vi "Sr830 Write Param.vi"(6 "Time Constant":u16(ring)=1 items=["10 us", "30 us", "100 us", "300 us", "1 ms", "3 ms", "10 ms", "30 ms", "100 ms", "300 ms", "1 s", "3 s", "10 s", "30 s", "100 s", "300 s", "1 ks", "3 ks", "10 ks", "30 ks"], 7 "Dynamic Reserve":u16(ring) items=["High", "Normal", "Low"], 8 "error in":errorcluster, 9 "Sensitivity":u16(ring)=1 items=["2 nV/fA", "5 nV/fA", "10 nV/fA", "20 nV/fA", "50 nV/fA", "100 nV/fA", "200 nV/fA", "500 nV/fA", "1 µV/pA", "2 µV/pA", "5 µV/pA", "10 µV/pA", "20 µV/pA", "50 µV/pA", "100µV/pA", "200 µV/pA", "500µV/pA", "1 mV/nA", "2 mV/nA", "5 mV/nA", "10 mV/nA", "20 mV/nA", "50 mV/nA", "100 mV/nA", "200 mV/nA", "500 mV/nA", "1 V/uA"], 10 "Param":T1(ring), 11 "Ressource VISA":refnum<visa-resource-name>="GPIB0::8::INSTR") -> (0 "error out":errorcluster, 3 "Ressource VISA Out":refnum<visa-resource-name>="GPIB0::8::INSTR")   [LabVIEW 2019]
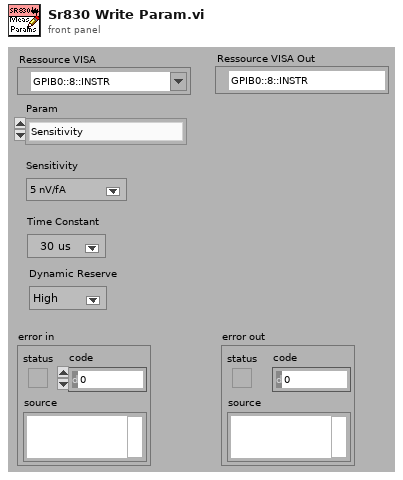
[diagram p1: front panel]
types:
  T1 = enum16{"Sensitivity", "Dynamic Reserve", "Time Constant"}
  T2 = enum16{"Phase Shift", "Reference Source", "Reference Frequency", "Reference Trigger", "Detection Harmonic", "Sine Amplitude", "Input Configuration", "Input Shield", "Input Coupling", "Input Line Notch Filter", "Sensitivity", "Dynamic Reserve", "Time Constant", "Low Pass Filter", "Sync Filter", "Expand X", "Expand Y", "Expand R", "All"}
  T3 = cluster{"Phase Shift (°)":dbl, "Reference Source":u16, "Frequency (Hz)":dbl, "Reference Trigger":u16, "Harmonic":i32, "Sine Amplitude (V)":dbl, "Input Configuration":u16, "Input Shield":u16, "Input Coupling":u16, "Input Notch Filters":cluster{"1xLineFilter":bool, "2xLineFilter":bool}, "Sensitivity":u16, "Dynamic Reserve":u16, "Time Constant":u16, "Low Pass Filter":u16, "Sync Filter":bool, "Expand X":cluster{"Offset (%)":dbl, "Expand":u16}, "Expand Y":cluster{"Offset (%)":dbl, "Expand":u16}, "Expand R":cluster{"Offset (%)":dbl, "Expand":u16}}
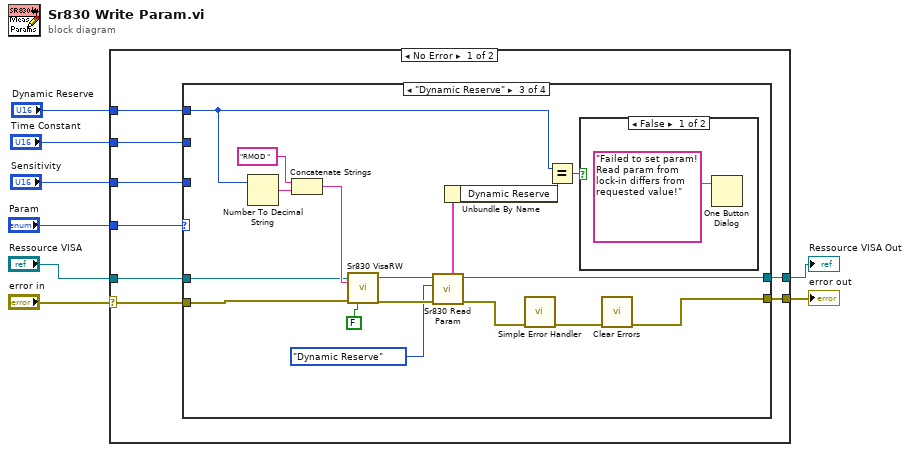
[diagram p0: block diagram]
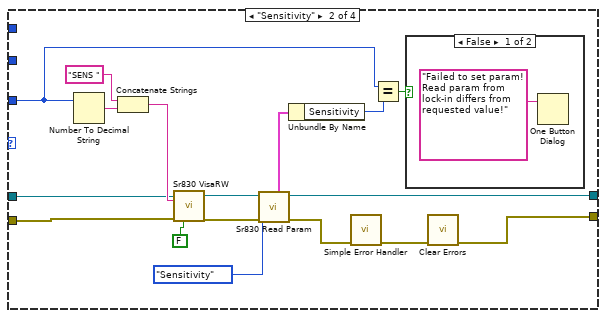
[diagram p3: hidden frame]
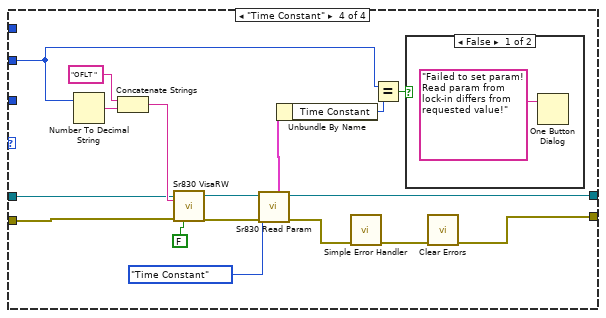
[diagram p6: hidden frame]
diagram:
  n1 = case shown="No Error" "error in" {
    selector: "error in" -> [w14 w74]
    tunnel: [w15 w74] -> w8
    tunnel: "Ressource VISA" -> [w13 w73]
    tunnel: [w16 w73] -> w5
    tunnel: "Sensitivity" -> [w12 _]
    tunnel: "Param" -> [w11 _]
    tunnel: "Dynamic Reserve" -> [w10 _]
    tunnel: "Time Constant" -> [w9 _]
    frame No Error {
      n2 = case shown="\"Dynamic Reserve\"" w11 {
        tunnel: [w17 w21 w40 w58] -> w16
        tunnel: [w18 w19 w38 w56] -> w15
        tunnel: w14 -> [w18 w31 w49 w67]
        tunnel: w13 -> [w17 w30 w48 w66]
        tunnel: w12 -> [_ w23 _ _]
        tunnel: w10 -> [_ _ w37 _]
        tunnel: w9 -> [_ _ _ w55]
        frame Default {
        }
        frame "Sensitivity" {
          n3 = Number To Decimal String(number=w23) -> (decimal integer string=w34:string)  [unwired: 1 in]
          n4 = Concatenate Strings("SENS " ("ChaineCom"), w34) -> (w32:string)
          n5 = call <userlib>:"Sr830 VisaRW.vi"("VISA Rsrc"=w30, "ChaineCom"=w32, "error in (no error)"=w31, "Lecture?(T)"=FALSE) -> ("VISA Rsrc Out"=w29:refnum<visa-resource-name>, "error out"=w28:errorcluster)  [unwired: 8 in, 2 out]
          n6 = call <userlib>:"Sr830 Read Param.vi"("error in (no error)"=w28, "Énum"=T2."Sensitivity", "Ressource VISA"=w29) -> ("error out"=w25:errorcluster, "Ressource VISA Out"=w21:refnum<visa-resource-name>, "LockInPar"=w26:T3)  [unwired: 5 in, 1 out]
          n7 = Unbundle By Name(w26) -> ("Sensitivity"=w24:u16)
          n8 = call <vilib>:"Simple Error Handler.vi"("error in (no error)"=w25) -> ("error out"=w20:errorcluster)  [unwired: 4 in, 4 out]
          n9 = Equal?(x=w23, y=w24) -> (x = y?=w22:bool)
          n10 = case shown="False" w22 {
            frame False {
              n11 = One Button Dialog(message="Failed to set param! Read param from lock-in differs from requested value!") -> ()  [unwired: 1 in, 1 out]
            }
            frame True {
            }
          }
          n12 = call <vilib>:"Clear Errors.vi"("error in (no error)"=w20) -> ("error out"=w19:errorcluster)  [unwired: 5 in, 1 out]
        }
        frame "Dynamic Reserve" {
          n13 = Number To Decimal String(number=w37) -> (decimal integer string=w52:string)  [unwired: 1 in]
          n14 = Concatenate Strings("RMOD " ("ChaineCom"), w52) -> (w50:string)
          n15 = call <userlib>:"Sr830 VisaRW.vi"("VISA Rsrc"=w48, "ChaineCom"=w50, "error in (no error)"=w49, "Lecture?(T)"=FALSE) -> ("VISA Rsrc Out"=w47:refnum<visa-resource-name>, "error out"=w46:errorcluster)  [unwired: 8 in, 2 out]
          n16 = call <userlib>:"Sr830 Read Param.vi"("error in (no error)"=w46, "Énum"=T2."Dynamic Reserve", "Ressource VISA"=w47) -> ("error out"=w43:errorcluster, "Ressource VISA Out"=w40:refnum<visa-resource-name>, "LockInPar"=w44:T3)  [unwired: 5 in, 1 out]
          n17 = Unbundle By Name(w44) -> ("Dynamic Reserve"=w42:u16)
          n18 = call <vilib>:"Simple Error Handler.vi"("error in (no error)"=w43) -> ("error out"=w39:errorcluster)  [unwired: 4 in, 4 out]
          n19 = Equal?(x=w37, y=w42) -> (x = y?=w41:bool)
          n20 = case shown="False" w41 {
            frame False {
              n21 = One Button Dialog(message="Failed to set param! Read param from lock-in differs from requested value!") -> ()  [unwired: 1 in, 1 out]
            }
            frame True {
            }
          }
          n22 = call <vilib>:"Clear Errors.vi"("error in (no error)"=w39) -> ("error out"=w38:errorcluster)  [unwired: 5 in, 1 out]
        }
        frame "Time Constant" {
          n23 = Number To Decimal String(number=w55) -> (decimal integer string=w70:string)  [unwired: 1 in]
          n24 = Concatenate Strings("OFLT " ("ChaineCom"), w70) -> (w68:string)
          n25 = call <userlib>:"Sr830 VisaRW.vi"("VISA Rsrc"=w66, "ChaineCom"=w68, "error in (no error)"=w67, "Lecture?(T)"=FALSE) -> ("VISA Rsrc Out"=w65:refnum<visa-resource-name>, "error out"=w64:errorcluster)  [unwired: 8 in, 2 out]
          n26 = call <userlib>:"Sr830 Read Param.vi"("error in (no error)"=w64, "Énum"=T2."Time Constant", "Ressource VISA"=w65) -> ("error out"=w61:errorcluster, "Ressource VISA Out"=w58:refnum<visa-resource-name>, "LockInPar"=w62:T3)  [unwired: 5 in, 1 out]
          n27 = Unbundle By Name(w62) -> ("Time Constant"=w60:u16)
          n28 = call <vilib>:"Simple Error Handler.vi"("error in (no error)"=w61) -> ("error out"=w57:errorcluster)  [unwired: 4 in, 4 out]
          n29 = Equal?(x=w55, y=w60) -> (x = y?=w59:bool)
          n30 = case shown="False" w59 {
            frame False {
              n31 = One Button Dialog(message="Failed to set param! Read param from lock-in differs from requested value!") -> ()  [unwired: 1 in, 1 out]
            }
            frame True {
            }
          }
          n32 = call <vilib>:"Clear Errors.vi"("error in (no error)"=w57) -> ("error out"=w56:errorcluster)  [unwired: 5 in, 1 out]
        }
      }
    }
    frame Error {
    }
  }
  "error out" <- w8
  "Ressource VISA Out" <- w5
